vi "Relay Set (Water Tank).vi"(8 "error in (no error)":errorcluster, 10 "RelayValue":enum16{"Off", "On"}(ring), 11 "RelayDevRef":cluster{string, i32}) -> (0 "error out":errorcluster, 3 "RelayDevRef":cluster{string, i32})   [LabVIEW 2013]
uses:
  Water Tank Global.vi
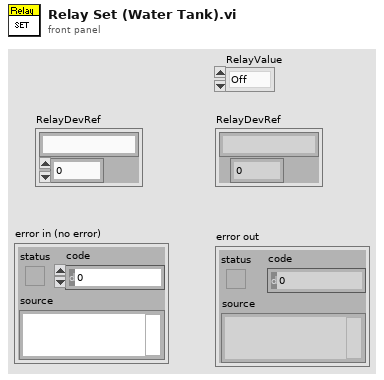
[diagram p1: front panel]
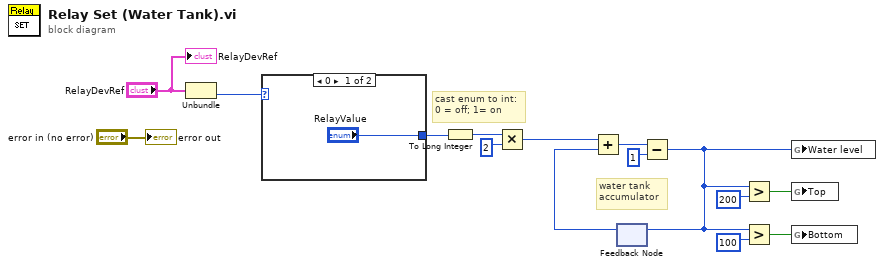
[diagram p0: block diagram]
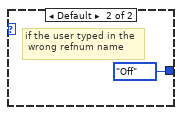
[diagram p2: hidden frame]
diagram:
  # "cast enum to int:\n0 = off; 1= on"
  # "water tank\naccumulator"
  n1 = Unbundle("RelayDevRef") -> (w13:i32)  [unwired: 1 out]
  n2 = case shown="0" w13 {
    tunnel: ["RelayValue" enum16{"Off", "On"}."Off" ("RelayValue")] -> w12
    frame 0 {
    }
    frame Default {
      # "if the user typed in the\n wrong refnum name"
    }
  }
  n3 = To Long Integer(number=w12) -> (32bit integer=w11:i32)
  n4 = Multiply(x=w11, y=2) -> (x*y=w9:i32)
  n5 = feedback #1() -> (w8:i32)  [unwired: 1 in]
  n6 = Add(x=w9, y=w8) -> (x+y=w3:i32)
  n7 = Subtract(x=w3, y=1) -> (x-y=w1:i32)
  n8 = feedback-in #1(w1) -> ()
  n9 = Greater?(x=w1, y=200) -> (0:w5:bool)
  n10 = Greater?(x=w1, y=100) -> (0:w4:bool)
  n11 = global write "Water Tank Global.vi" "Water level"(w1) -> ()
  n12 = global write "Water Tank Global.vi" "Top"(w5) -> ()
  n13 = global write "Water Tank Global.vi" "Bottom"(w4) -> ()
  "error out" <- "error in (no error)"
  "RelayDevRef" <- "RelayDevRef"
